vi "SignalGenerator.vi"(4 "error in":errorcluster caption="error in (no error)", 5 "stop":bool, 6 "Frequency":dbl, 7 "Amplitude":dbl) -> (0 "error out":errorcluster)   [LabVIEW 2014]
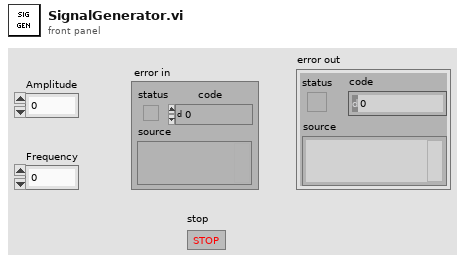
[diagram p1: front panel]
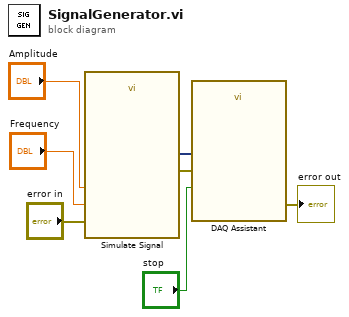
[diagram p0: block diagram]
diagram:
  n1 = call "Simulate Signal"("Frequency"="Frequency", "Amplitude"="Amplitude", "error in (no error)"="error in") -> ("Sine"=w7:dynamicdata, "error out"=w6:errorcluster)  [unwired: 11 in]
  n2 = call "DAQ Assistant"("data"=w7, "error in"=w6, "stop (F)"="stop") -> ("error out"=→"error out":errorcluster)  [unwired: 14 in, 2 out]
